vi "GetWindowHandle.vi"(11 "Window in":refnum<class "Window.lvclass">) -> (2 "SDL_Window *":i64, 3 "Window out":refnum<class "Window.lvclass">)   [LabVIEW 2024, in "GLF.lvlib" / "Window.lvclass"]
uses:
  Window.lvclass
  Window.lvclass/Window.ctl
  95d46fde-ebac-4d2f-abc6-cfa2c877d26e.vi
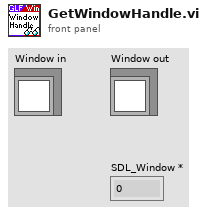
[diagram p1: front panel]
types:
  T1 = typedef "GLF.lvlib/Window.lvclass/DVR--cluster.ctl" = cluster{"SDL_Window *":i64}
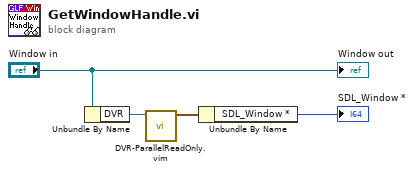
[diagram p0: block diagram]
diagram:
  n1 = Unbundle By Name("Window in") -> ("DVR"=w3:refnum<data-value>)
  n2 = call "DVR-ParallelReadOnly.vim"("DVR"=w3) -> ("Data"=w2:T1)  [unwired: 9 in, 1 out]
  n3 = Unbundle By Name(w2) -> ("SDL_Window *"=→"SDL_Window *":i64)
  "Window out" <- "Window in"
